vi "SetAnalogOutput.vi"(0 "controller in":refnum<k24>, 5 "axis name":string, 7 "port":i32 min=0 max=2 step=1, 9 "value":dbl min=0.0 max=255.0 step=1.0, 11 "error in (no error)":errorcluster) -> (4 "controller out":refnum<k24>, 15 "error out":errorcluster)   [LabVIEW 2010]
uses:
  c:/aerotech/controller/5.xx.xxx/ensemble/pc/labview/2010/bin/Aerotech.Ensemble.dll
  bin/Aerotech.Ensemble.dll
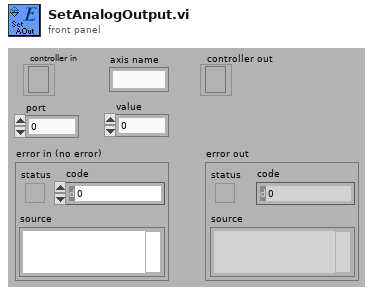
[diagram p1: front panel]
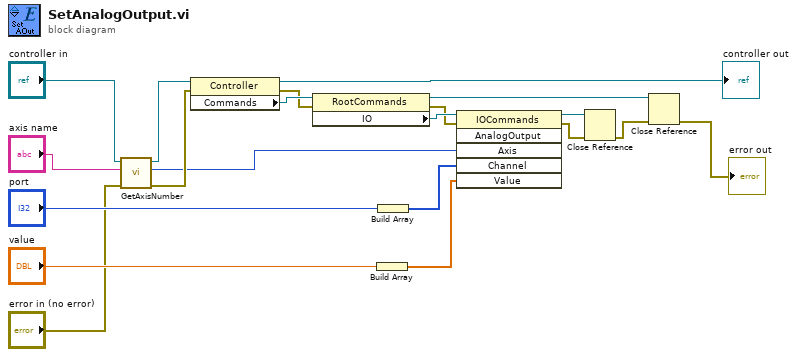
[diagram p0: block diagram]
diagram:
  n1 = call "GetAxisNumber.vi"("error in (no error)"="error in (no error)", "axis name"="axis name", "controller in"="controller in") -> ("error out"=w13:errorcluster, "axis number"=w8:i32, "controller out"=w11:refnum<k24>)  [unwired: 6 in]
  n2 = property class="Controller"(reference=w11, error in=w13) -> (reference out=→"controller out":refnum<k24>, error out=w18:errorcluster, "Commands"=w19:refnum<k24>)
  n3 = property class="RootCommands"(reference=w19, error in=w18) -> (reference out=w3:refnum<k24>, error out=w16:errorcluster, "IO"=w17:refnum<k24>)
  n4 = Build Array("value") -> (w6:dbl[])
  n5 = Build Array("port") -> (w7:i32[])
  n6 = invoke class="IOCommands" method="AnalogOutput"(reference=w17, error in=w16, "Axis"=w8, "Channel"=w7, "Value"=w6) -> (reference out=w4:refnum<k24>, error out=w5:errorcluster)  [unwired: 1 in, 4 out]
  n7 = Close Reference(reference=w4, error in (no error)=w5) -> (error out=w2:errorcluster)
  n8 = Close Reference(reference=w3, error in (no error)=w2) -> (error out=→"error out":errorcluster)
